vi "ShooterRangeCompensation.vi"(1 "Range Delay (s)":dbl, 2 "Fused Distance to Target (in)":dbl) -> (0 "Adjusted Distance to Target (in)":dbl)   [LabVIEW 2020]
uses:
  sensordata.vi
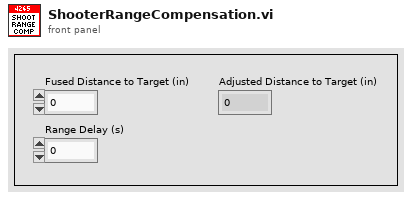
[diagram p1: front panel]
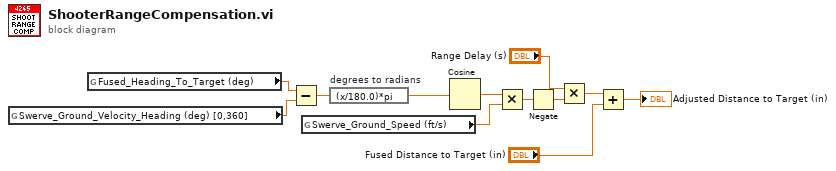
[diagram p0: block diagram]
diagram:
  n1 = global read "sensordata.vi" "Swerve_Ground_Velocity_Heading (deg) [0,360]"() -> (w4:dbl)
  n2 = global read "sensordata.vi" "Fused_Heading_To_Target (deg)"() -> (w3:dbl)
  n3 = Subtract(x=w3, y=w4) -> (x-y=w5:dbl)
  n4 = global read "sensordata.vi" "Swerve_Ground_Speed (ft/s)"() -> (w8:dbl)
  n5 = expression code="(x/180.0)*pi" "degrees to radians"(w5) -> (w6:dbl)
  n6 = Cosine(x=w6) -> (cos(x)=w7:dbl)
  n7 = Multiply(x=w7, y=w8) -> (x*y=w9:dbl)
  n8 = Negate(x=w9) -> (-x=w10:dbl)
  n9 = Multiply(x="Range Delay (s)", y=w10) -> (x*y=w12:dbl)
  n10 = Add(x=w12, y="Fused Distance to Target (in)") -> (x+y=→"Adjusted Distance to Target (in)":dbl)
